vi "_save_csv_SingleSweep.vi"(7 "delimiter (\\t)":string="SingleCh_", 11 "Data":dbl[][](array[numeric])) -> (3 "FileName":string)   [LabVIEW 2023]
uses:
  <vilib>/Utility/file.llb/Write Delimited Spreadsheet (string).vi
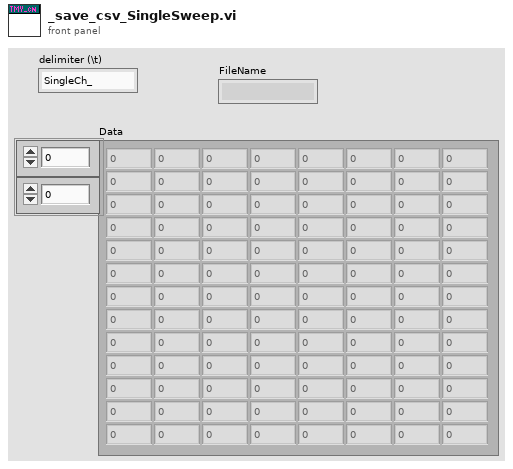
[diagram p1: front panel]
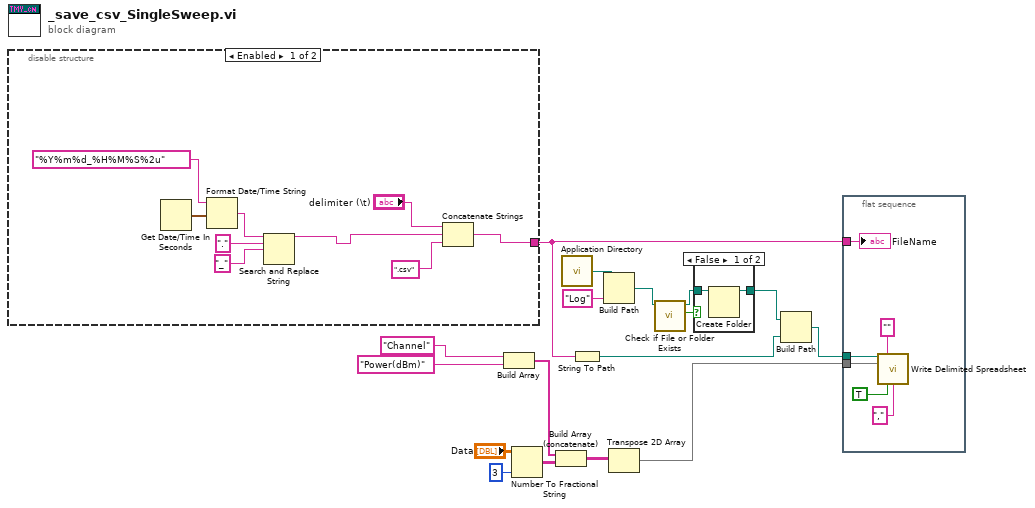
[diagram p0: block diagram]
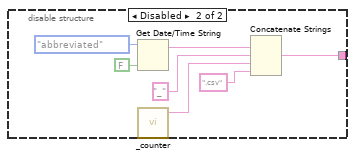
[diagram p3: hidden frame]
diagram:
  n1 = disable-structure shown="Enabled" {
    disable-tunnel: [w25 w27] -> w14
    frame Enabled {
      n2 = Get Date/Time In Seconds() -> (seconds since 1Jan1904=w23:timestamp)
      n3 = Format Date/Time String(time format string (%c)="%Y%m%d_%H%M%S%2u", seconds (now)=w23) -> (date/time string=w21:string)  [unwired: 1 in]
      n4 = Search and Replace String(input string=w21, search string=".", replace string="_") -> (result string=w18:string)  [unwired: 5 in, 3 out]
      n5 = Concatenate Strings("delimiter (\\t)", w18, ".csv" ("delimiter (\\t)")) -> (w25:string)
    }
    frame Disabled {
      n6 = Get Date/Time String(date format (0)=enum16{"short", "long", "abbreviated"}."abbreviated", want seconds? (F)=FALSE) -> (date string=w34:string)  [unwired: 1 in, 1 out]
      n7 = call "_counter.vi"() -> ("out_count"=w28:string)  [unwired: 5 in]
      n8 = Concatenate Strings(w34, "_" ("delimiter (\\t)"), w28, ".csv" ("delimiter (\\t)")) -> (w27:string, w29:string)
    }
  }
  n9 = Build Array("Channel", "Power(dBm)") -> (w3:string[])
  n10 = Number To Fractional String(number="Data", precision (6)=i16 3) -> (F-format string=w4:string[][])  [unwired: 2 in]
  n11 = Build Array (concatenate)(w3, w4) -> (w2:string[][])
  n12 = call <vilib>:"Application Directory.vi"() -> ("Application Directory"=w13:path)
  n13 = String To Path(string=w14) -> (path=w16:path)
  n14 = Build Path(base path=w13, name or relative path="Log") -> (appended path=w10:path)
  n15 = Transpose 2D Array(2D array=w2) -> (transposed array=w1:string[][])
  n16 = call <vilib>:"Check if File or Folder Exists.vi"("path"=w10) -> ("file or folder exists?"=w12:bool, "dup path"=w11:path)  [unwired: 8 in, 1 out]
  n17 = case shown="False" w12 {
    tunnel: w11 -> [w36 w37]
    tunnel: [w35 w37] -> w9
    frame False {
      n18 = Create Folder(path (use dialog)=w36) -> (created path=w35:path)  [unwired: 2 in, 2 out]
    }
    frame True {
    }
  }
  n19 = Build Path(base path=w9, name or relative path=w16) -> (appended path=w15:path)
  n20 = flat-sequence {
    tunnel: w15 -> [w42]
    tunnel: w14 -> [w40]
    tunnel: w1 -> [w38]
    frame #0 {
      n21 = call-poly <vilib>:"Write Delimited Spreadsheet.vi"("file path (dialog if empty)"=w42, "format (%s)"="" ("format (%.3f)"), "2D data"=w38, "transpose? (no:F)"=TRUE, "delimiter (\\t)"="," ("delimiter (\\t)")) -> ()  [unwired: 9 in, 2 out]
      "FileName" <- w40
    }
  }
